vi "hum_filter.vi"(5 "Noise limit":bool, 7 "Reset":bool, 9 "Input":dbl[](array[numeric]), 10 "Config":T2={"I/O"={"Buffering (in/out)"=[], "Output Device"=0, "Sound"={"sample rate (S/s)"=0.0, "number of channels"=0, "bits per sample"=0}, "Input Device"=0}, "Noise limit low"=0.0, "Distortion LF cut"=0.0, "Averaging Tc"=0.0, "High rate STFT"={"Win param"=101.5, "Window type"=61, "Win order"=2, "DFT size"=64, "Channels"=[7], "Oversample"=64}, "Low rate STFT"={"Win param"=120.0, "Window type"=61, "Win order"=8, "DFT size"=64, "Channels"=[7], "Oversample"=64}, "Hum filter"={"Frequency"=0.0, "Tc"=0.0}} {"Low rate STFT"."Oversample" min=1 step=1; "Low rate STFT"."Channels" min=0 step=1; "Low rate STFT"."DFT size" min=1 step=1; "Low rate STFT"."Window type" items=["Rectangle"=0, "Hanning"=1, "Hamming"=2, "Blackman-Harris"=3, "Exact Blackman"=4, "Blackman"=5, "Flat Top"=6, "4 Term B-Harris "=7, "7 Term B-Harris"=8, "Low Sidelobe"=9, "Blackman Nuttall"=11, "Triangle"=30, "Bartlett-Hanning"=31, "Bohman"=32, "Parzen"=33, "Welch"=34, "Kaiser"=60, "Dolph-Chebyshev"=61, "Gaussian"=62]; "High rate STFT"."Oversample" min=1 step=1; "High rate STFT"."Channels" min=0 step=1; "High rate STFT"."DFT size" min=1 step=1; "High rate STFT"."Window type" items=["Rectangle"=0, "Hanning"=1, "Hamming"=2, "Blackman-Harris"=3, "Exact Blackman"=4, "Blackman"=5, "Flat Top"=6, "4 Term B-Harris "=7, "7 Term B-Harris"=8, "Low Sidelobe"=9, "Blackman Nuttall"=11, "Triangle"=30, "Bartlett-Hanning"=31, "Bohman"=32, "Parzen"=33, "Welch"=34, "Kaiser"=60, "Dolph-Chebyshev"=61, "Gaussian"=62]; "I/O"."Input Device" format="%.0x"; "I/O"."Output Device" format="%.0x"}, 11 "Modulation info":T1 {"Hi channels at low" min=0 step=1; "Low carriers" format="%#_6p"; "High carriers" format="%#_6p"}) -> (0 "Hum variance (synch)":dbl[](array[numeric]), 1 "Hum (synch)":dbl[](array[numeric]), 2 "Hum variance":dbl[](array[numeric]), 3 "Hum":dbl[](array[numeric]))   [LabVIEW 2014]
uses:
  <vilib>/sound2/lvsound2.llb/Sound Data Format.ctl
  <vilib>/Analysis/4window.llb/windowTd.ctl
  <vilib>/Analysis/NI_AALPro.lvlib
  stft_params.ctl
  ilemt_config.ctl
  modulation_info.ctl
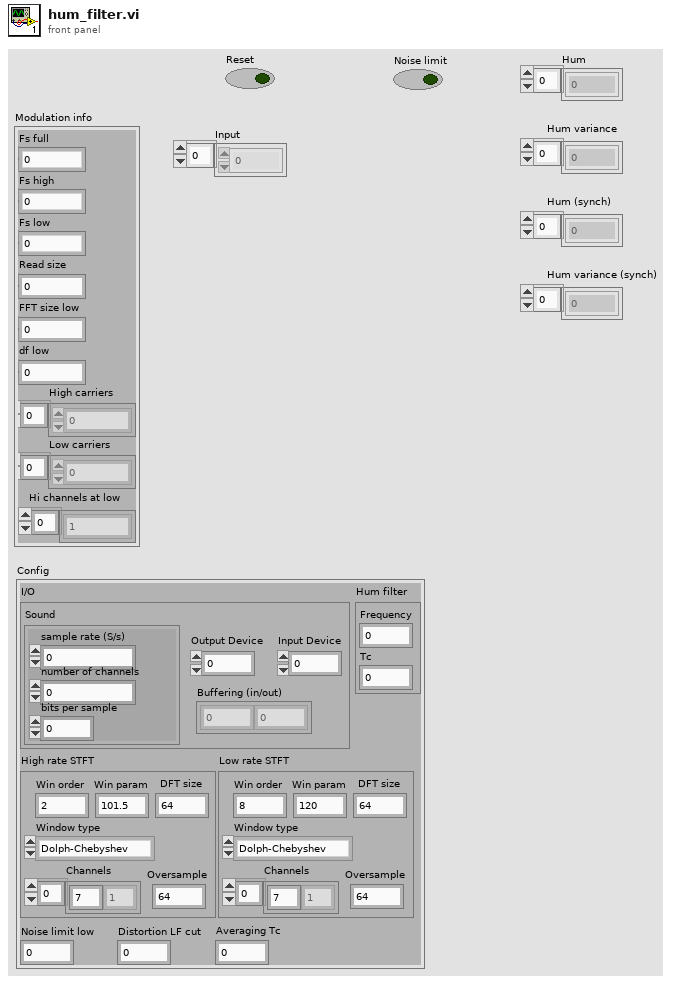
[diagram p1: front panel]
types:
  T1 = typedef "modulation_info.ctl" = cluster{"Fs full":dbl, "Fs high":dbl, "Fs low":dbl, "Read size":i32, "FFT size low":i32, "df low":dbl, "High carriers":dbl[], "Low carriers":dbl[], "Hi channels at low":i32[]}
  T2 = typedef "ilemt_config.ctl" = cluster{"I/O":cluster{"Buffering (in/out)":dbl[], "Output Device":u32, "Sound":T3, "Input Device":u32}, "Noise limit low":dbl, "Distortion LF cut":dbl, "Averaging Tc":sgl, "High rate STFT":T4, "Low rate STFT":T4, "Hum filter":cluster{"Frequency":dbl, "Tc":dbl}}
  T3 = typedef "Sound Data Format.ctl" = cluster{"sample rate (S/s)":dbl, "number of channels":i32, "bits per sample":i32}
  T4 = typedef "stft_params.ctl" = cluster{"Win param":dbl, "Window type":T5, "Win order":i32, "DFT size":i32, "Channels":i32[], "Oversample":i32}
  T5 = typedef "NI_AALPro.lvlib/windowTd.ctl" = u32
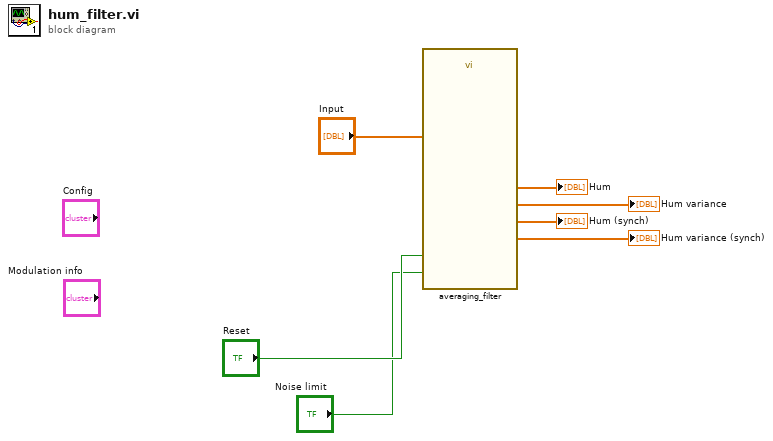
[diagram p0: block diagram]
diagram:
  n1 = call "averaging_filter.vi"(4:"Noise limit", "Reset"="Reset", "Input"="Input") -> ("Order variance"=→"Hum variance (synch)":dbl[], "Order mean"=→"Hum (synch)":dbl[], "Variance"=→"Hum variance":dbl[], "Mean"=→"Hum":dbl[], "Order"=w6:i32, "Time constant (samples)"=w5:dbl)  [unwired: 3 in]
